vi "RFM Control and Status.Get Register Offset.vi"(11 "RFM Control and Status Register":T1) -> (3 "Offset":u32)   [LabVIEW 2016, in "GE 5565PIORC.lvclass"]
uses:
  GE 5565PIORC.lvclass
  Controls/Registers.RFM Control and Status.ctl
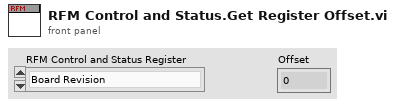
[diagram p1: front panel]
types:
  T1 = typedef "GE 5565PIORC.lvclass/Registers.RFM Control and Status.ctl" = enum16{"Board Revision", "Board ID", "Board Revision Build", "Node ID", "Local Control and Status", "Local Interrupt Status", "Local Interrupt Enable", "Network Target Data", "Network Target Node", "Network Interrupt Command", "Interrupt 1 Sender Data", "Interrupt 1 Sender ID", "Interrupt 2 Sender Data", "Interrupt 2 Sender ID", "Interrupt 3 Sender Data", "Interrupt 3 Sender ID", "Interrupt 4 Sender Data", "Interrupt 4 Sender ID"}
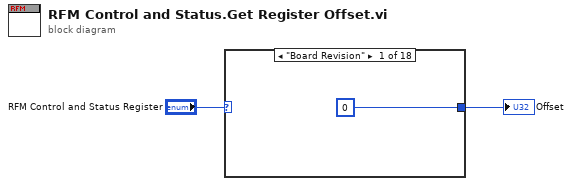
[diagram p0: block diagram]
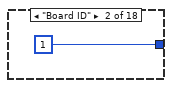
[diagram p2: hidden frame]
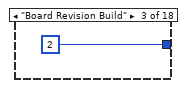
[diagram p3: hidden frame]
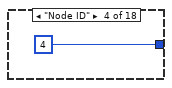
[diagram p4: hidden frame]
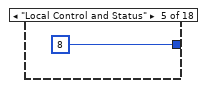
[diagram p5: hidden frame]
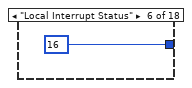
[diagram p6: hidden frame]
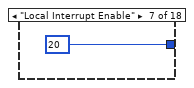
[diagram p7: hidden frame]
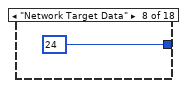
[diagram p8: hidden frame]
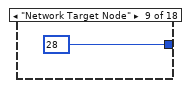
[diagram p9: hidden frame]
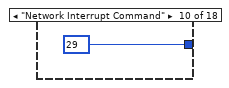
[diagram p10: hidden frame]
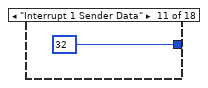
[diagram p11: hidden frame]
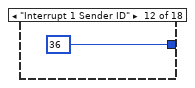
[diagram p12: hidden frame]
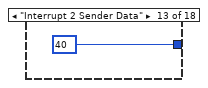
[diagram p13: hidden frame]
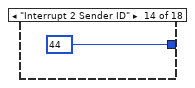
[diagram p14: hidden frame]
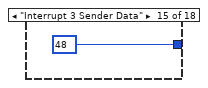
[diagram p15: hidden frame]
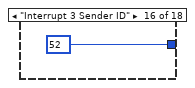
[diagram p16: hidden frame]
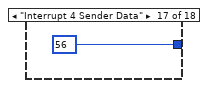
[diagram p17: hidden frame]
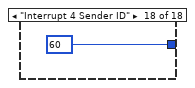
[diagram p18: hidden frame]
diagram:
  n1 = case shown="\"Board Revision\"" "RFM Control and Status Register" {
    tunnel: [u32 0 u32 1 u32 2 u32 4 u32 8 u32 16 u32 20 u32 24 u32 28 u32 29 u32 32 u32 36 u32 40 u32 44 u32 48 u32 52 u32 56 u32 60] -> w2
    frame "Board Revision" {
    }
    frame "Board ID" {
    }
    frame "Board Revision Build" {
    }
    frame "Node ID" {
    }
    frame "Local Control and Status" {
    }
    frame "Local Interrupt Status" {
    }
    frame "Local Interrupt Enable" {
    }
    frame "Network Target Data" {
    }
    frame "Network Target Node" {
    }
    frame "Network Interrupt Command" {
    }
    frame "Interrupt 1 Sender Data" {
    }
    frame "Interrupt 1 Sender ID" {
    }
    frame "Interrupt 2 Sender Data" {
    }
    frame "Interrupt 2 Sender ID" {
    }
    frame "Interrupt 3 Sender Data" {
    }
    frame "Interrupt 3 Sender ID" {
    }
    frame "Interrupt 4 Sender Data" {
    }
    frame "Interrupt 4 Sender ID" {
    }
  }
  "Offset" <- w2
